vi "Login_to_webserver_invalid_password.vi"() -> ()   [LabVIEW 2017]
uses:
  Generic_Common/Webserver/html_report_cluster.ctl
  <vilib>/httpClient/LabVIEWHTTPClient.lvlib
panel:
  out "StatusCodeName":string
  out "Session id name":string
  out "logout_url":string
  out "ErrorCode_expected":string
  out "Logout : Header  debug purpose":string
  out "Logout : Body debug purpose":string
  out "Status_message":string
  out "Logo":u16(ring)
  out "Iteration_Indicator":dbl
  out "Error code recieved":i32
  out "POST_command":string
  out "Command_url":string
  out "Test case":string
  out "Global ini path":path
  out "Test status":picture
  out "Time elapsed for each iteration":string
  out "DelayBetweenIterations":string
  out "Total_Iterations":i32
  out "Global_Webserver_Report":string
  out "TestSuite":string
  out "Error Out":errorcluster
  out "Response time":u32[](graph)
  out "Header of reponse for debug pupose":string
  out "Response from the web server":string
  # "AUTOMATION TESTING WEB SERVICES"
  # "TESTING DETAILS FROM INI"
  # "RESPONSE FROM WEBSERVER"
  # "ms"
  # "Webserver \n1. Webserver is being tested in this test case where SC board of ultrasonic welding machine is connected to test PC \t\t  \nSC IP address: 192.168.2.101, url=https://192.168.2.101\t\t\t\t\t\t\t\t\t\t \t\t\t  \n2. Ports used on SC board are as below:\t\t\t\t\t\t\t\t\t\t\t\t\t\t\t\t\t\t\t\t\t  \n   - J103: (Ethernet0) This port connected to UI controller large screen HMI display\trestricted webservices in this port\t\t\t\t\t\t\t\t\t  \n  - J104: (Ethernet1) This port is connected to local area network for accessing the webpage and testing  webserver                                \n  - J112: SC Logs are taken from this port. TeraTerm is configured  to this port so that SC logs are displayed on the screen."
  # "ms"
  # "Debug purpose"
  # "RESPONSE TIME GRAPH"
  # "TESTING STATUS"
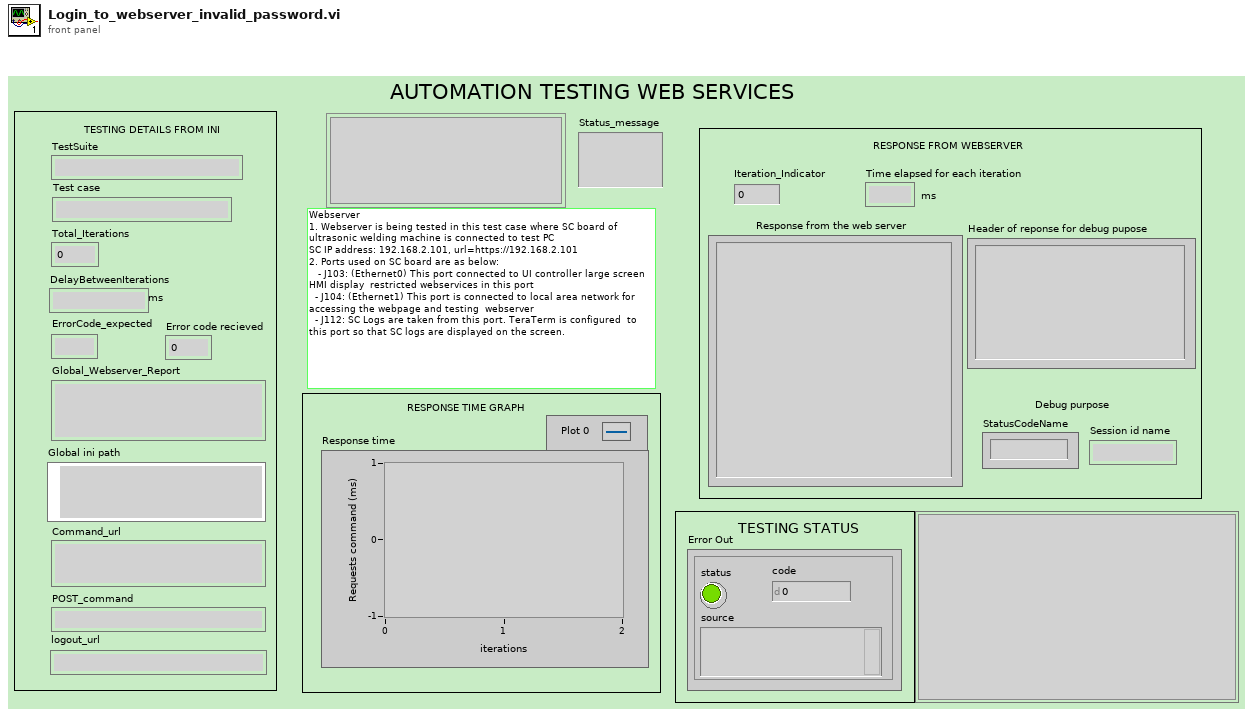
[diagram p1: front panel]
types:
  T1 = enum16{"open", "replace", "create", "open or create", "replace or create", "replace or create with confirmation"}
  T2 = enum8{"Enabled", "Disabled", "Disabled and Grayed Out"}
  T3 = cluster{"[0]":string, "[1]":string, "[2]":string, "[3]":string, "[4]":string, "[5]":string, "[6]":string, "[7]":string, "[8]":string}
  T4 = cluster{"login_url":string, "userid":string, "password":string, "key":string, "command_url":string, "POST_command":string, "StatusCode_expected":string, "Iterations":string, "DelayBetweenIterations":string, "Timeout":string, "logout_url":string, "TestSuite":string}
  T5 = cluster{"Server_IP_Address":string, "Server_Port_Number":string, "Sid":string, "StatusCodeName":string, "Global_Webserver_Report":string}
  T6 = typedef "html_report_cluster.ctl" = cluster{"Remarks":string, "Verdict":string, "Status Code":i32, "Status Description":string, "JazzDashboardLink":string, "ReprtPath":string, "Timestamp":string, "TestSuite":string, "TestCase":string, "Iterations":i64, "Time taken to execute  test in msec":string, "Delay Between Iterations":i64}
  T7 = typedef "LabVIEWHTTPClient.lvlib/ClientHandle.ctl" = refnum<k1>
  T8 = typedef "imagedata.ctl" = cluster{"image type":i32, "image depth":i32, "image":u8[], "mask":u8[], "colors":u32[], "Rectangle":cluster{"left":i16, "top":i16, "right":i16, "bottom":i16}}
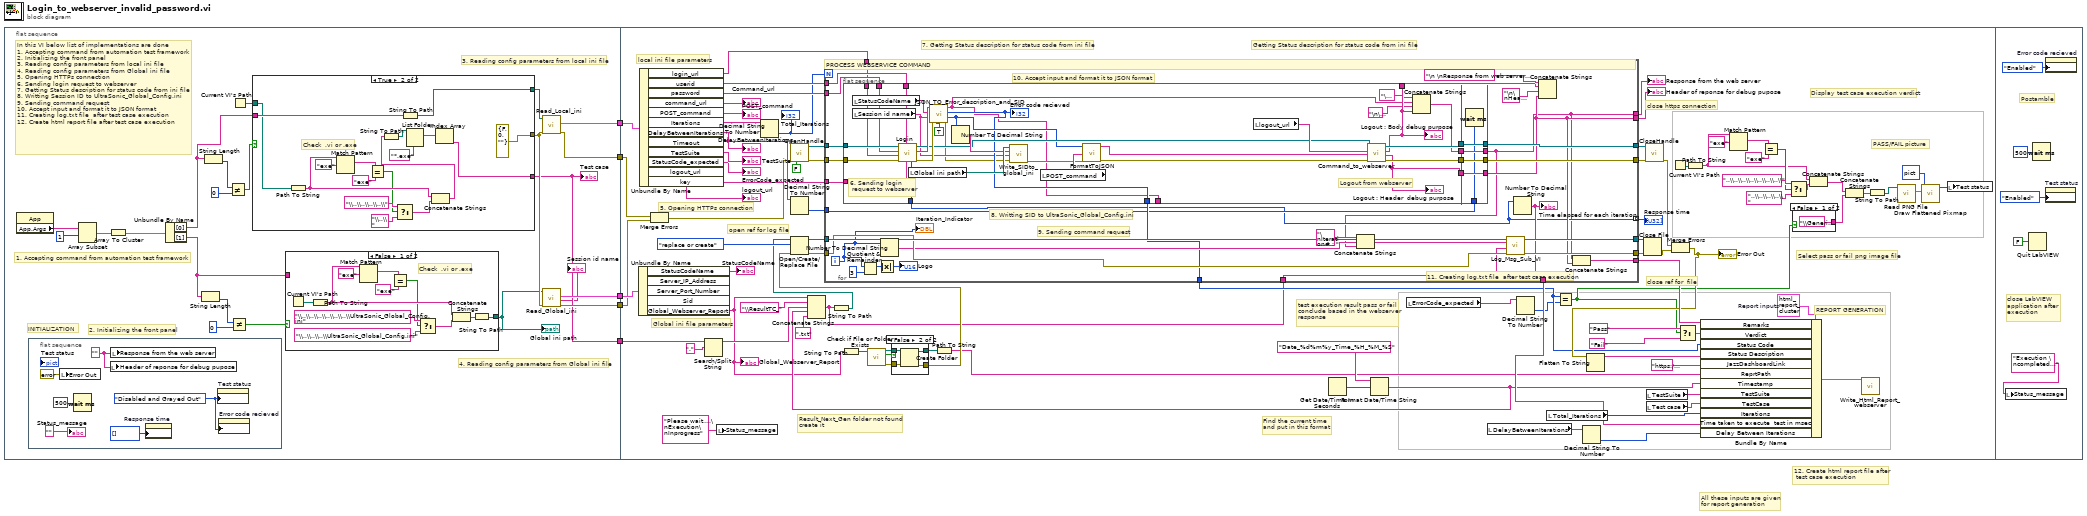
[diagram p0: block diagram]
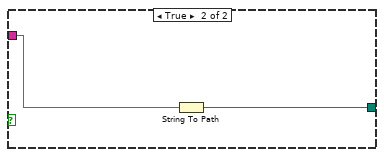
[diagram p2: hidden frame]
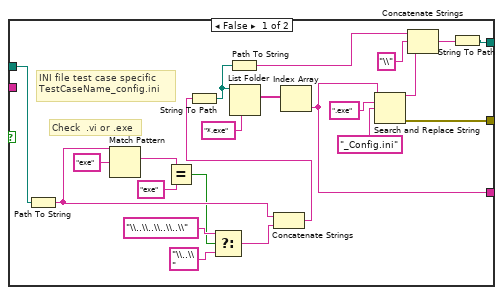
[diagram p3: hidden frame]
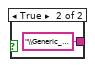
[diagram p5: hidden frame]
diagram:
  # "All these inputs are given \nfor report generation"
  # "12. Create html report file after\n test case execution"
  n1 = flat-sequence {
    tunnel: [w16] -> w5
    tunnel: [w19] -> w4
    tunnel: [w18] -> w3
    tunnel: [w17] -> w2
    tunnel: [w7] -> w1
    tunnel: w5 -> [w140]
    tunnel: w4 -> [w172]
    tunnel: w3 -> [w173]
    tunnel: w2 -> [w139]
    tunnel: w1 -> [w112]
    frame #0 {
      # "INITIALIZATION"
      # "4. Reading config parameters from Global ini file"
      # "3. Reading config parameters from local ini file"
      # "2. Initializing the front panel"
      # "1. Accepting command from automation test framework"
      # "In this VI below list of implementations are done\n1. Accepting command from automation test framework\n2. Initializing the front panel\n3. Reading config parameters from local ini file\n4. Reading config parameters from Global ini file\n5. Opening HTTPs connection\n6. Sending login request to webserver\n7. Getting Status description for status code from ini file\n8. Writting Session ID to UltraSonic_Global_Config.ini\n9. Sending command request\n10. Accept input and format it to JSON format\n11. Creating log.txt file  after test case execution\n12. Create html report file after test case execution"
      n2 = property class="App"() -> ("App.Args"=w21:string[])  [unwired: 2 in, 2 out]
      n3 = flat-sequence {
        frame #0 {
          w28 = T2."Disabled and Grayed Out" ("Disabled")
          w33 = ""
          n4 = local write "Error Out"(errorcluster {"status"=FALSE, "code"=0, "source"=""} ("error constant")) -> ()
          n5 = Wait (ms)(milliseconds to wait=u32 500) -> ()  [unwired: 1 out]
          n6 = local write "Header of reponse for debug pupose"(w33) -> ()
          n7 = local write "Response from the web server"(w33) -> ()
          n8 = property on="Response time" class="WFChart (strict)"("History Data"=u32[] []) -> ()  [unwired: 2 in, 2 out]
          n9 = property on="Test status" class="Pict"("DisabledEnum"=w28) -> ()  [unwired: 2 in, 2 out]
          n10 = property on="Error code recieved" class="DigNum (strict)"("DisabledEnum"=w28) -> ()  [unwired: 2 in, 2 out]
          "Status_message" <- ""
        }
      }
      n11 = Array Subset "Array Subset"(array=w21, index=1) -> (w22:string[])  [unwired: 1 in]
      n12 = Array To Cluster(array=w22) -> (cluster=w23:T3)
      n13 = Unbundle By Name "Unbundle By Name"(w23) -> ("[0]"=w15:string, "[1]"=w10:string)
      n14 = String Length(string=w10) -> (length=w27:i32)
      n15 = String Length(string=w15) -> (length=w24:i32)
      n16 = Not Equal?(x=w24, y=0) -> (x != y?=w13:bool)
      n17 = Not Equal?(x=w27, y=0) -> (x != y?=w11:bool)
      n18 = Current VI's Path() -> (path=w14:path)
      n19 = case shown="True" w13 {
        tunnel: w15 -> [_ w85]
        tunnel: [w61 w84] -> w8
        tunnel: [w60 errorcluster {"status"=FALSE, "code"=0, "source"=""} ("error out")] -> w12
        tunnel: w14 -> [w49 w70]
        tunnel: [w47 w69] -> w7
        frame False {
          # "Check  .vi or .exe"
          # "INI file test case specific\nTestCaseName_config.ini"
          n20 = Path To String(path=w49) -> (string=w54:string)
          n21 = Match Pattern(string=w54, regular expression="exe") -> (match substring=w53:string)  [unwired: 1 in, 3 out]
          n22 = Equal?(x=w53, y="exe") -> (x = y?=w51:bool)
          n23 = Select(t="\\..\\..\\..\\..\\" ("string"), s=w51, f="\\..\\" ("string")) -> (s? t:f=w55:string)
          n24 = Concatenate Strings(w54, w55) -> (w48:string)
          n25 = String To Path(string=w48) -> (path=w59:path)
          n26 = Path To String(path=w59) -> (string=w58:string)
          n27 = List Folder(path=w59, pattern="*.exe") -> (filenames=w62:string[])  [unwired: 2 in, 3 out]
          n28 = Index Array(array=w62) -> (element=w47:string)  [unwired: 1 in]
          n29 = Search and Replace String(input string=w47, search string=".exe", replace string="_Config.ini" ("replace string (\"\")")) -> (result string=w66:string, error out=w60:errorcluster)  [unwired: 5 in, 2 out]
          n30 = Concatenate Strings(w58, "\\" ("string"), w66) -> (w64:string)
          n31 = String To Path(string=w64) -> (path=w61:path)
        }
        frame True {
          # "Check  .vi or .exe"
          n32 = Path To String(path=w70) -> (string=w76:string)
          n33 = Match Pattern(string=w76, regular expression="exe") -> (match substring=w75:string)  [unwired: 1 in, 3 out]
          n34 = Equal?(x=w75, y="exe") -> (x = y?=w73:bool)
          n35 = Select(t="\\..\\..\\..\\..\\" ("string"), s=w73, f="\\..\\" ("string")) -> (s? t:f=w77:string)
          n36 = String To Path(string=w85) -> (path=w84:path)
          n37 = Concatenate Strings(w76, w77) -> (w71:string)
          n38 = String To Path(string=w71) -> (path=w80:path)
          n39 = List Folder(path=w80, pattern="*.exe") -> (filenames=w81:string[])  [unwired: 2 in, 3 out]
          n40 = Index Array(array=w81) -> (element=w69:string)  [unwired: 1 in]
        }
      }
      "Test case" <- w7
      n41 = case shown="False" w11 {
        tunnel: [w43 w46] -> w9
        tunnel: w10 -> [_ w45]
        frame False {
          # "Check  .vi or .exe"
          n42 = Current VI's Path() -> (path=w35:path)
          n43 = Path To String(path=w35) -> (string=w39:string)
          n44 = Match Pattern(string=w39, regular expression="exe") -> (match substring=w38:string)  [unwired: 1 in, 3 out]
          n45 = Equal?(x=w38, y="exe") -> (x = y?=w36:bool)
          n46 = Select(t="\\..\\..\\..\\..\\..\\..\\UltraSonic_Global_Config.ini" ("string"), s=w36, f="\\..\\..\\..\\UltraSonic_Global_Config.ini" ("string")) -> (s? t:f=w40:string)
          n47 = Concatenate Strings(w39, w40) -> (w44:string)
          n48 = String To Path(string=w44) -> (path=w43:path)
        }
        frame True {
          n49 = String To Path(string=w45) -> (path=w46:path)
        }
      }
      "Global ini path" <- w9
      n50 = call "Read_Local_ini.vi"("Error In"=w12, "Local ini path"=w8) -> ("Error Out"=w16:errorcluster, "Read from ini file"=w18:T4)  [unwired: 8 in]
      n51 = call "Read_Global_ini.vi"("Error In"=w12, "Global ini path"=w9) -> ("Error Out"=w17:errorcluster, "Session id name"=→"Session id name":string, "Global Cluster"=w19:T5)  [unwired: 7 in]
    }
    frame #1 {
      w155 = T6 {"Remarks"="", "Verdict"="", "Status Code"=0, "Status Description"="", "JazzDashboardLink"="", "ReprtPath"="", "Timestamp"="", "TestSuite"="", "TestCase"="", "Iterations"=0, "Time taken to execute  test in msec"="", "Delay Between Iterations"=1000}  # Report inputs
      # "Getting Status description for status code from ini file"
      # "7. Getting Status description for status code from ini file"
      # "Select pass or fail png image file"
      # "test execution result pass or fail\nconclude based in the webserver\nresponse"
      # "Find the current time \nand put in this format"
      # "open ref for log file"
      # "Result_Next_Gen folder not found\ncreate it"
      # "Global ini file parameters"
      # "local ini file parameters"
      # "close ref for  file"
      # "close https connection"
      # "Display test case execution verdict"
      # "11. Creating log.txt file  after test case execution"
      # "5. Opening HTTPs connection"
      # "REPORT GENERATION"
      # "PASS/FAIL picture"
      n52 = Unbundle By Name(w172) -> ("StatusCodeName"=→"StatusCodeName":string, "Global_Webserver_Report"=w104:string)  [unwired: 3 out]
      "Global_Webserver_Report" <- w104
      n53 = Unbundle By Name(w173) -> ("login_url"=w135:string, "userid"=w169:string, "password"=w168:string, "command_url"=→"Command_url":string, "POST_command"=→"POST_command":string, "Iterations"=w165:string, "DelayBetweenIterations"=w164:string, "TestSuite"=→"TestSuite":string, "StatusCode_expected"=→"ErrorCode_expected":string, "logout_url"=→"logout_url":string, "key"=w86:string)  [unwired: 1 out]
      "DelayBetweenIterations" <- w164
      n54 = Merge Errors(w140, w139) -> (w138:errorcluster)
      n55 = Search/Split String(string=w112, search string/char (-)=".") -> (substring before match=w110:string)  [unwired: 1 in, 2 out]
      n56 = local write "Status_message"("Please wait....\nExecution\nInprogress") -> ()
      n57 = Decimal String To Number(string=w165) -> (number=w153:i32)  [unwired: 2 in, 1 out]
      "Total_Iterations" <- w153
      n58 = call <vilib>:"OpenHandle.vi"("error in (no error)"=w138, "verify server(true)"=FALSE) -> ("client handle out"=w171:T7, "error out"=w170:errorcluster)  [unwired: 12 in]
      n59 = Decimal String To Number(string=w164) -> (number=w163:i32)  [unwired: 2 in, 1 out]
      n60 = String To Path(string=w104) -> (path=w109:path)
      n61 = call <vilib>:"Check if File or Folder Exists.vi"("path"=w109) -> ("error out"=w105:errorcluster, "file or folder exists?"=w108:bool, "dup path"=w107:path)  [unwired: 8 in]
      n62 = case shown="False" w108 {
        tunnel: [w174 w179] -> w103
        tunnel: w107 -> [w175 w178]
        tunnel: [w175 w177] -> w106
        tunnel: w105 -> [w174 w176]
        frame True {
        }
        frame False {
          n63 = Create Folder(path (use dialog)=w178, error in=w176) -> (created path=w177:path, error out=w179:errorcluster)  [unwired: 1 in, 1 out]
        }
      }
      n64 = Path To String(path=w106) -> (string=w102:string)
      n65 = Get Date/Time In Seconds() -> (seconds since 1Jan1904=w90:timestamp)
      n66 = Format Date/Time String(time format string (%c)="Date_%d%m%y_Time_%H_%M_%S", seconds (now)=w90) -> (date/time string=w115:string)  [unwired: 1 in]
      n67 = Concatenate Strings(w104, "\\ResultTC_" ("string"), w110, w115, ".txt" ("string")) -> (w89:string)
      n68 = String To Path(string=w89) -> (path=w113:path)
      n69 = Open/Create/Replace File(file path (use dialog)=w113, error in=w103, operation (0:open)=T1."replace or create") -> (refnum out=w162:refnum<file>, error out=w161:errorcluster)  [unwired: 3 in, 1 out]
      n70 = for {
        N: w153 -> [_]
        tunnel: w171 -> [w215]
        tunnel: w168 -> [w212]
        tunnel: [w183] -> w167
        tunnel: w169 -> [w213]
        tunnel: [w197] -> w166
        tunnel: w170 -> [w214]
        tunnel: w163 -> [w190]
        tunnel: [w184] -> w146 mode=indexing
        tunnel: w162 -> [w210]
        tunnel: w161 -> [w209]
        tunnel: [w208] -> w160
        tunnel: [w207] -> w159
        tunnel: [w203] -> w157
        tunnel: [w202] -> w156
        tunnel: [w198] -> w144
        tunnel: w135 -> [w200]
        tunnel: [w196] -> w117
        tunnel: [w191] -> w95
        tunnel: w89 -> [w185]
        tunnel: w86 -> [w182]
        i -> [w193]
        # "8. Writting SID to UltraSonic_Global_Config.ini"
        # "10. Accept input and format it to JSON format"
        # "9. Sending command request"
        # "PROCESS WEBSERVICE COMMAND"
        n71 = flat-sequence {
          tunnel: w213 -> [w244]
          tunnel: w212 -> [w243]
          tunnel: [w227] -> w189
          tunnel: [w226] -> w188
          tunnel: [w240] -> w187
          tunnel: [w239] -> w186
          tunnel: w200 -> [w242]
          tunnel: [w221] -> w199
          tunnel: [w225] -> w191
          tunnel: [w220] -> _
          tunnel: [w233] -> w184
          tunnel: w215 -> [w246]
          tunnel: w214 -> [w245]
          tunnel: w182 -> [w216]
          tunnel: [w248] -> w202
          tunnel: [w249] -> w203
          tunnel: [w250] -> w197
          tunnel: [w251] -> w183
          tunnel: w189 -> [w251]
          tunnel: w188 -> [w250]
          tunnel: w187 -> [w249]
          tunnel: w186 -> [w248]
          tunnel: w190 -> [w247]
          frame #0 {
            # "Logout from webserver"
            # "6. Sending login\n request to webserver"
            n72 = local read "StatusCodeName"() -> (w223:string)
            n73 = local read "Session id name"() -> (w222:string)
            n74 = call "Login.vi"("key"=w216, "userid"=w244, "Error In"=w245, "Command to webservice"=w242, "password"=w243, "IN HTTPS client handle"=w246) -> ("Error Out"=w235:errorcluster, "Body of reponse"=w232:string, "OUT HTTPS client handle"=w231:T7, "Response time"=w233:u32)  [unwired: 1 in, 1 out]
            n75 = local read "Global ini path"() -> (w238:path)
            n76 = call "JSON_TO_Error_description_and_SID.vi"("Sid_present_in_webserver_response"=TRUE, "Error In"=w235, "Session id name"=w222, "Status code name"=w223, "JSON String input"=w232) -> ("Error Out"=w217:errorcluster, "SID"=w228:i32, "status code"=w225:i32, "status_selected"=w220:string)  [unwired: 3 in]
            "Error code recieved" <- w225
            n77 = Number To Decimal String(number=w228) -> (decimal integer string=w236:string)  [unwired: 1 in]
            n78 = call "Write_SIDto_global_ini.vi"("Error In"=w217, "Session id name"=w222, "SID"=w236, "Global ini path"=w238) -> ("Error Out"=w237:errorcluster)  [unwired: 7 in]
            n79 = local read "POST_command"() -> (w241:string)
            n80 = call "FormatToJSON.vi"("Error In"=w237, "Post_command"=w241, "Sid"=w228) -> ("Error Out"=w230:errorcluster, "Final_POST_Command"=w229:string)  [unwired: 6 in, 1 out]
            n81 = local read "logout_url"() -> (w234:string)
            n82 = call "Command_to_webserver.vi"("Error In"=w230, "JSON post command"=w229, "URL Command to Logout"=w234, "https client handle in ref"=w231) -> ("Error Out"=w240:errorcluster, "Header of response for debug purpose"=w226:string, "Body of response"=w221:string, "https client handle out ref"=w239:T7)  [unwired: 3 in, 1 out]
            "Logout : Body debug purpose" <- w221
            "Logout : Header  debug purpose" <- w226
            n83 = Concatenate Strings("\nLogin:\n" ("string"), w220, "\n\nLogout:\n" ("string"), w221) -> (w227:string)
          }
          frame #1 {
            n84 = Wait (ms)(milliseconds to wait=w247) -> ()  [unwired: 1 out]
          }
        }
        n85 = Quotient & Remainder(x=w193, y=3) -> (x-y*floor(x/y)=w194:i32)  [unwired: 1 out]
        n86 = Absolute Value(x=w194) -> (abs(x)=→"Logo":i32)
        n87 = Number To Decimal String(number=w193) -> (decimal integer string=w204:string)  [unwired: 1 in]
        n88 = Concatenate Strings("\nIteration# : " ("string"), w204, w183) -> (w206:string)
        n89 = call "Log_Msg_Sub_VI.vi"("Error In"=w209, "Path for CSV"=w185, "String input"=w206, "refnum in"=w210) -> ("Error Out"=w207:errorcluster, "refnum out"=w208:refnum<file>)  [unwired: 6 in]
        n90 = Number To Decimal String(number=w184) -> (decimal integer string=w196:string)  [unwired: 1 in]
        "Time elapsed for each iteration" <- w196
        n91 = Concatenate Strings("\n \nResponse from web server# :\n" ("string"), w199, "\n\nHeader# : \n", w197) -> ()  [unwired: 1 out]
        n92 = Concatenate Strings(w183, w197) -> (w198:string)
        "Iteration_Indicator" <- w193
      }
      "Response from the web server" <- w167
      "Header of reponse for debug pupose" <- w166
      "Response time" <- w146
      n93 = local read "ErrorCode_expected"() -> (w96:string)
      n94 = local read "DelayBetweenIterations"() -> (w148:string)
      n95 = Decimal String To Number(string=w96) -> (number=w94:i32)  [unwired: 2 in, 1 out]
      n96 = local read "Total_Iterations"() -> (w149:i32)
      n97 = Equal?(x=w95, y=w94) -> (x = y?=w93:bool)
      n98 = Decimal String To Number(string=w148) -> (number=w147:i32)  [unwired: 2 in, 1 out]
      n99 = Close File(refnum=w160, error in=w159) -> (error out=w151:errorcluster)  [unwired: 1 out]
      n100 = call <vilib>:"CloseHandle.vi"("client handle"=w156, "error in (no error)"=w157) -> ("error out"=w152:errorcluster)  [unwired: 13 in]
      n101 = local read "TestSuite"() -> (w150:string)
      n102 = local read "Test case"() -> (w137:string)
      n103 = Current VI's Path() -> (path=w123:path)
      n104 = Merge Errors(w152, w151) -> (w101:errorcluster)
      "Error Out" <- w101
      n105 = Flatten To String(anything=w101) -> (data string=w100:string)  [unwired: 3 in, 2 out]
      n106 = Select(t="Pass", s=w93, f="Fail") -> (s? t:f=w141:string)
      n107 = Path To String(path=w123) -> (string=w121:string)
      n108 = Bundle By Name(cluster=w155, "Remarks"=w144, "Verdict"=w141, "Status Code"=w95, "Status Description"=w100, "JazzDashboardLink"="https://jazz.bucclm.com/", "ReprtPath"=w102, "Timestamp"=w115, "TestSuite"=w150, "TestCase"=w137, "Iterations"=w149, "Time taken to execute  test in msec"=w117, "Delay Between Iterations"=w147) -> (w154:T6)
      n109 = Match Pattern(string=w121, regular expression="exe") -> (match substring=w127:string)  [unwired: 1 in, 3 out]
      n110 = Equal?(x=w127, y="exe") -> (x = y?=w125:bool)
      n111 = Select(t="..\\..\\..\\..\\..\\..\\..\\" ("string"), s=w125, f="..\\..\\..\\..\\" ("string")) -> (s? t:f=w122:string)
      n112 = case shown="False" w93 {
        tunnel: ["\\Generic_Common\\\\Webserver\\\\Fail.png" "\\Generic_Common\\\\Webserver\\\\Pass.png"] -> w131
        frame False {
        }
        frame True {
        }
      }
      n113 = Concatenate Strings(w121, w122) -> (w120:string)
      n114 = Concatenate Strings(w120, w131) -> (w130:string)
      n115 = call "Write_Html_Report_webserver.vi"("Report inputs"=w154) -> ()  [unwired: 18 in, 1 out]
      n116 = String To Path(string=w130) -> (path=w119:path)
      n117 = call <vilib>:"Read PNG File.vi"("path to PNG file"=w119) -> ("image data"=w118:T8)  [unwired: 8 in, 2 out]
      n118 = call <vilib>:"Draw Flattened Pixmap.vi"("image data"=w118, "picture"=picture data[5B]) -> ("new picture"=w88:picture)  [unwired: 7 in]
      n119 = local write "Test status"(w88) -> ()
    }
    frame #2 {
      # "close LabVIEW \napplication after \nexecution"
      # "Postamble"
      n120 = local write "Status_message"("Execution \ncompleted...") -> ()
      n121 = Quit LabVIEW(quit? (T)=FALSE) -> ()
      n122 = Wait (ms)(milliseconds to wait=u32 500) -> ()  [unwired: 1 out]
      n123 = property on="Test status" class="Pict"("DisabledEnum"=T2."Enabled" ("Disabled")) -> ()  [unwired: 2 in, 2 out]
      n124 = property on="Error code recieved" class="DigNum (strict)"("DisabledEnum"=T2."Enabled" ("Disabled")) -> ()  [unwired: 2 in, 2 out]
    }
  }
